vi "Create ramping array.vi"(8 "Error In":errorcluster, 9 "Delta":dbl=0.5, 10 "End":dbl=3.0, 11 "Start":dbl=-3.0) -> (0 "Error Out":errorcluster, 2 "Array length":i32, 3 "Output Array (1D)":dbl[](array[numeric]))   [LabVIEW 2015]
uses:
  <vilib>/Utility/error.llb/Error Cluster From Error Code.vi
  <vilib>/ErrorRing/Error Ring.xnode
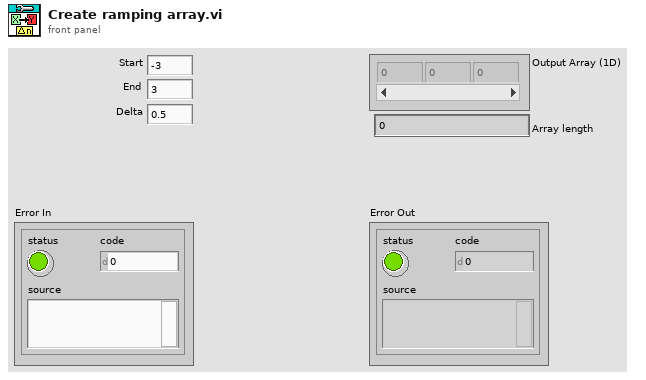
[diagram p1: front panel]
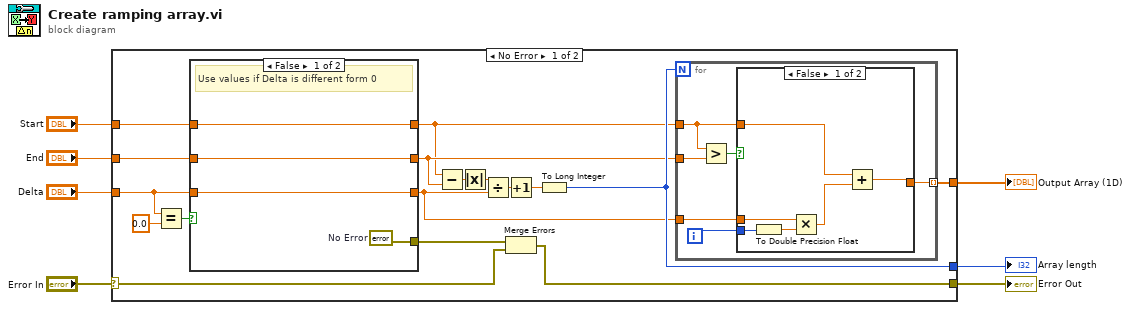
[diagram p0: block diagram]
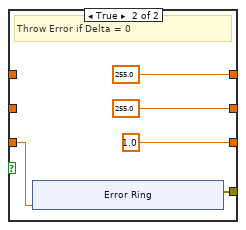
[diagram p2: hidden frame]
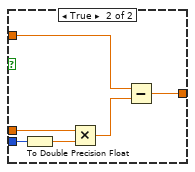
[diagram p3: hidden frame]
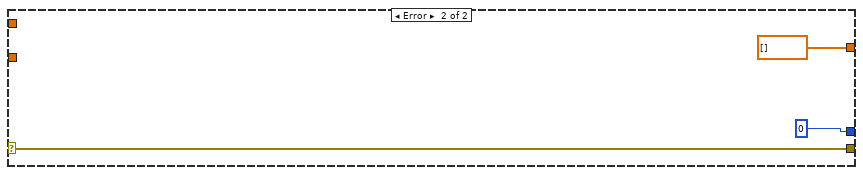
[diagram p4: hidden frame]
diagram:
  n1 = case shown="No Error" "Error In" {
    selector: "Error In" -> [w16 w61]
    tunnel: "End" -> [w12 _]
    tunnel: [w22 dbl[] []] -> w6
    tunnel: "Start" -> [w14 _]
    tunnel: "Delta" -> [w9 _]
    tunnel: [w15 w61] -> w2
    tunnel: [w19 0] -> w1
    frame No Error {
      n2 = Equal?(x=w9, y=0.0) -> (x = y?=w10:bool)
      n3 = case shown="False" w10 {
        tunnel: [w25 1.0] -> w18
        tunnel: [w26 w31] -> w17
        tunnel: [w27 255.0 ("Start")] -> w8
        tunnel: w14 -> [w27 _]
        tunnel: [w28 255.0 ("End")] -> w13
        tunnel: w12 -> [w28 _]
        tunnel: w9 -> [w25 w29]
        frame False {
          w26 = errorcluster {"status"=FALSE, "code"=0, "source"=""}  # No Error
          # "Use values if Delta is different form 0"
        }
        frame True {
          # "Throw Error if Delta = 0"
          n4 = xnode "Error Ring"("parameter 0"=w29) -> ("error out"=w31:errorcluster)
        }
      }
      n5 = Subtract(x=w8, y=w13) -> (x-y=w24:dbl)
      n6 = Absolute Value(x=w24) -> (abs(x)=w23:dbl)
      n7 = Divide(x=w23, y=w18) -> (x/y=w21:dbl)
      n8 = Increment(x=w21) -> (x+1=w20:dbl)
      n9 = Merge Errors(w17, w16) -> (w15:errorcluster)
      n10 = To Long Integer(number=w20) -> (32bit integer=w19:i32)
      n11 = for {
        N: w19 -> [_]
        tunnel: w8 -> [w45]
        tunnel: w13 -> [w44]
        tunnel: [w42] -> w22 mode=indexing
        tunnel: w18 -> [w41]
        i -> [w43]
        n12 = Greater?(x=w45, y=w44) -> (0:w46:bool)
        n13 = case shown="False" w46 {
          tunnel: w45 -> [w49 w55]
          tunnel: w43 -> [w48 w54]
          tunnel: w41 -> [w52 w58]
          tunnel: [w50 w56] -> w42
          frame False {
            n14 = To Double Precision Float(number=w48) -> (double precision float=w47:dbl)
            n15 = Multiply(x=w52, y=w47) -> (x*y=w51:dbl)
            n16 = Add(x=w49, y=w51) -> (x+y=w50:dbl)
          }
          frame True {
            n17 = To Double Precision Float(number=w54) -> (double precision float=w53:dbl)
            n18 = Multiply(x=w58, y=w53) -> (x*y=w57:dbl)
            n19 = Subtract(x=w55, y=w57) -> (x-y=w56:dbl)
          }
        }
      }
    }
    frame Error {
    }
  }
  "Array length" <- w1
  "Output Array (1D)" <- w6
  "Error Out" <- w2
